vi "SudokuSolver.vi"() -> ()   [LabVIEW 2020]
panel:
  out "Status":bool
  out "Error out":string
  in  "Solve with Matlab":bool
  out "Picture":picture
  in  "Jpeg path":path
  # "OCR Sudoku solver"
  # "Programmation pour ingénieur - Projet 2021"
  # "Images are expected as 400 x 400 JPG, with Helvetica font"
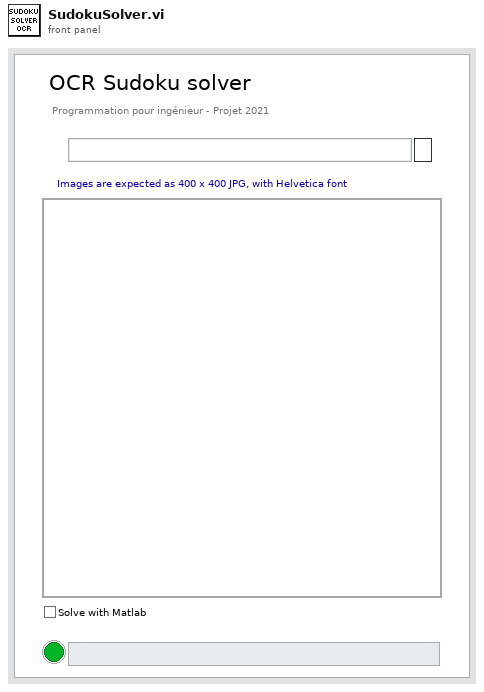
[diagram p1: front panel]
types:
  T1 = typedef "imagedata.ctl" = cluster{"image type":i32, "image depth":i32, "image":u8[], "mask":u8[], "colors":u32[], "Rectangle":cluster{"left":i16, "top":i16, "right":i16, "bottom":i16}}
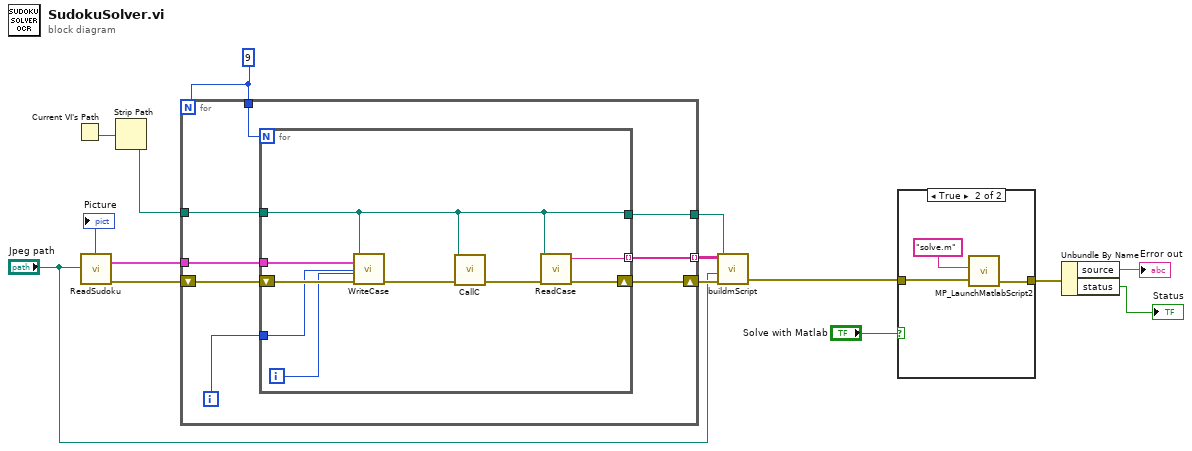
[diagram p0: block diagram]
diagram:
  w10 = 9
  n1 = Current VI's Path() -> (path=w15:path)
  n2 = call "ReadSudoku.vi"("Jpeg path"="Jpeg path") -> ("error out"=w13:errorcluster, "image data"=w12:T1, "Picture"=→"Picture":picture)  [unwired: 8 in]
  n3 = Strip Path(path=w15) -> (stripped path=w11:path)  [unwired: 1 out]
  n4 = for {
    N: w10 -> [_]
    tunnel: w12 -> [w21]
    tunnel: w11 -> [w20]
    tunnel: [w19] -> w9 mode=indexing
    shift-right: [w23] -> w8
    shift-left: w13 -> [w22]
    tunnel: w10 -> [w17]
    tunnel: [w16] -> w6
    i -> [w18]
    n5 = for {
      N: w17 -> [_]
      tunnel: w21 -> [w28]
      tunnel: w20 -> [w24]
      tunnel: [w27] -> w19 mode=indexing
      shift-right: [w32] -> w23
      shift-left: w22 -> [w30]
      tunnel: w18 -> [w26]
      tunnel: [w24] -> w16
      i -> [w25]
      n6 = call "WriteCase.vi"("Iteration 1st loop"=w26, "error in (no error)"=w30, "Iteration 2nd loop"=w25, "image data"=w28, "appended path"=w24) -> ("error out"=w29:errorcluster)  [unwired: 6 in]
      n7 = call "CallC.vi"("error in (no error)"=w29, "stripped path"=w24) -> ("error out"=w31:errorcluster)  [unwired: 9 in]
      n8 = call "ReadCase.vi"("error in (no error)"=w31, "stripped path"=w24) -> ("error out"=w32:errorcluster, "text"=w27:string)  [unwired: 8 in]
    }
  }
  n9 = call "buildmScript.vi"("error in (no error)"=w8, "Jpeg path"="Jpeg path", "Input array"=w9, "Current path"=w6) -> ("error out"=w4:errorcluster)  [unwired: 7 in]
  n10 = case shown="True" "Solve with Matlab" {
    tunnel: w4 -> [w33 w36]
    tunnel: [w33 w35] -> w3
    frame False {
    }
    frame True {
      n11 = call "MP_LaunchMatlabScript2.vi"("error in (no error)"=w36, "matlab script name with extension"="solve.m") -> ("error out"=w35:errorcluster)  [unwired: 5 in, 4 out]
    }
  }
  n12 = Unbundle By Name(w3) -> ("source"=→"Error out":string, "status"=→"Status":bool)
